vi "ServerGlobalVariables.vi"() -> ()   [LabVIEW 2025]
panel:
  out "Round":u32=1
  in  "Game State":T1(ring)
  in  "FieldArray":T2(array[cluster])
  in  "PlayerColorArray":u32[](array[colorbox])=[16711680, 2593535, 32768, 32896, 16419841, 15741670, 8388736, 10158337, 11775026, 10116644, 1061375, 5852325, 8759580, 16737896, 11829194, 11835761]
  in  "Options":map{string, u32}(c390)
  in  "Teams":set{u32}[](array[numeric])
  in  "Empty Team Slots":set{u8}(c389)
  in  "PlayerInfoMap":T3(c390)
  in  "PlayerIDConnectionMap":map{u32, cluster{"Address":u32, "Port":u16}}(c390)
  in  "PlayerConnectionIDMap":map{cluster{"Address":u32, "Port":u16}, u32}(c390)
  out "ID Counter":u32=1
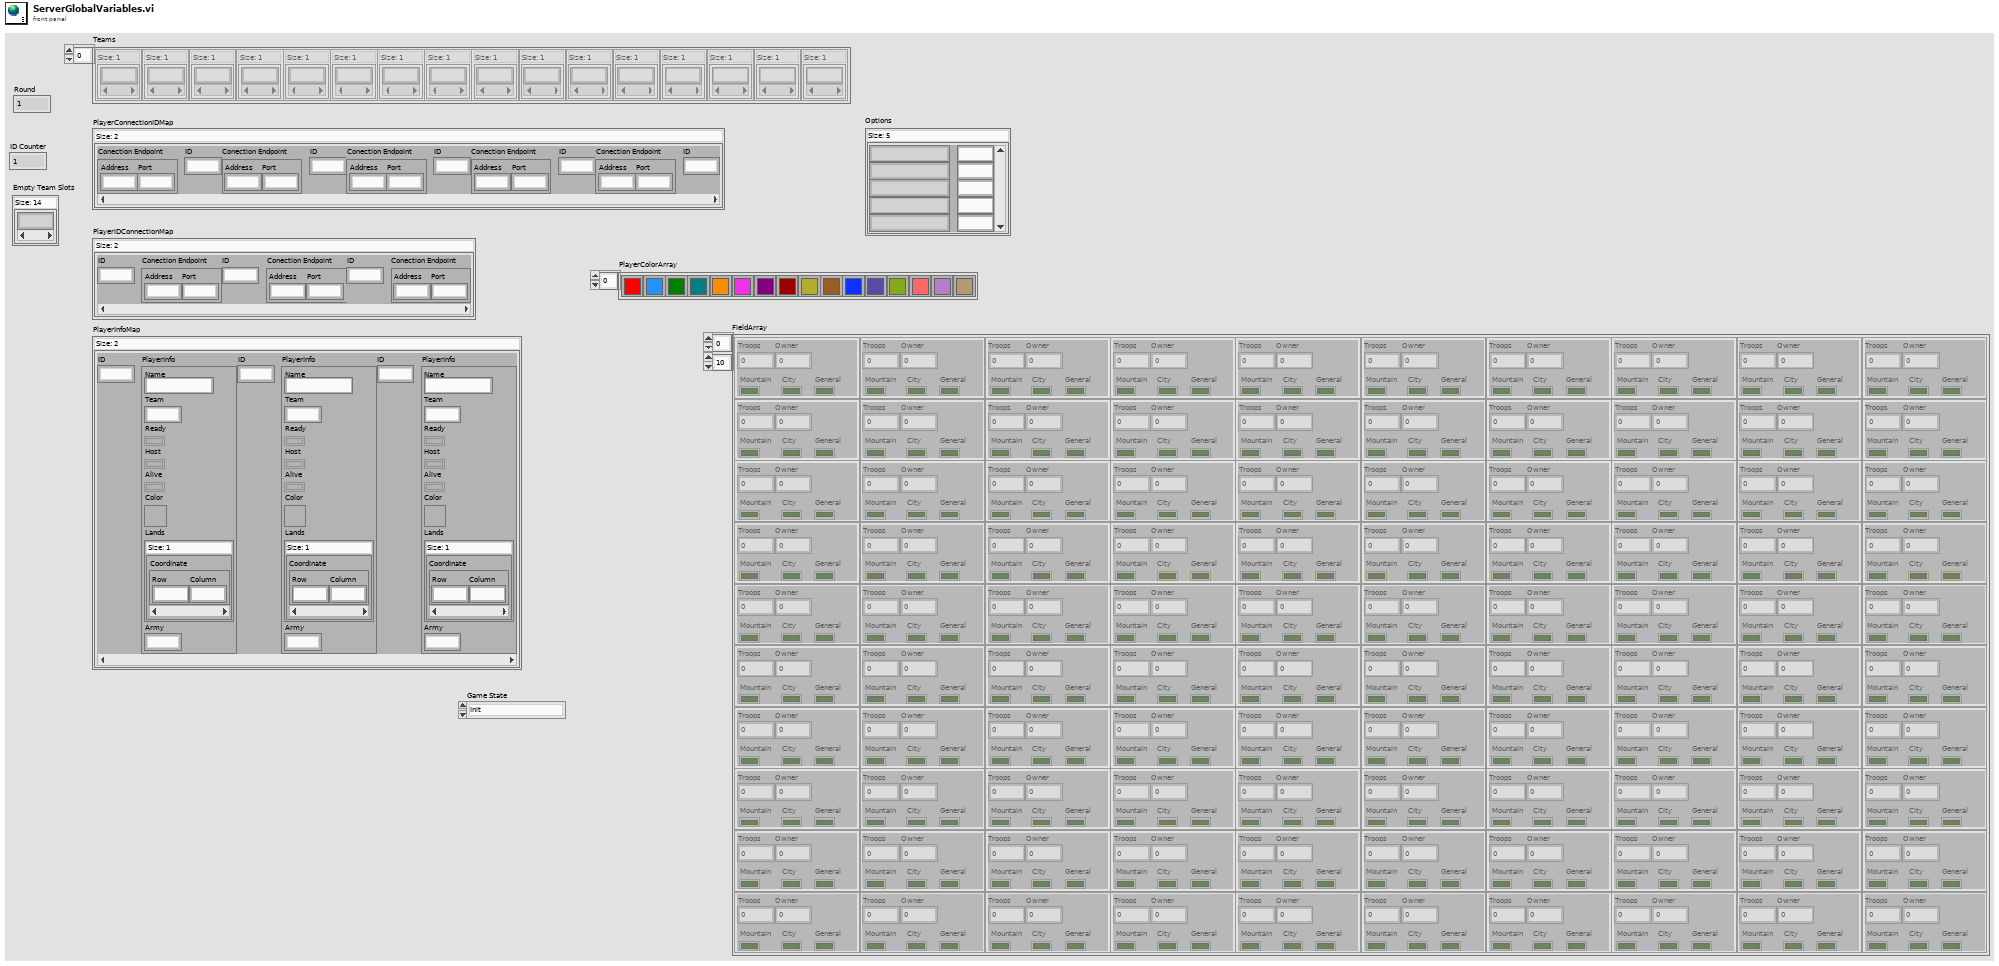
[diagram p1: front panel]
types:
  T1 = enum16{"Init", "Lobby", "Game Init", "Game", "Game End"}
  T2 = cluster{"Troops":u32, "Owner":i32, "Mountain":bool, "City":bool, "General":bool}[][]
  T3 = map{u32, cluster{"Name":string, "Team":u8, "Ready":bool, "Host":bool, "Alive":bool, "Color":u32, "Lands":set{cluster{"Row":u32, "Column":u32}}, "Army":u32}}
diagram:
